vi "attributes2Variant.vi"(0 "HGF_DIMBaseType":refnum<class "HGF_DIMDataConverter.lvclass">, 2 "Parameter":variant, 3 "typeDescriptor":string, 5 "error in (no error)":errorcluster) -> (14 "HGF_DIMBaseType":refnum<class "HGF_DIMDataConverter.lvclass">, 16 "rawData":variant, 19 "error out":errorcluster)   [LabVIEW 2012, in "HGF_DIM.lvlib" / "HGF_DIMDataConverter.lvclass"]
doc: "Convert variant attributes Pn, n=0,1,2,... to raw data value of variant."
uses:
  HGF_DIMDataConverter.lvclass
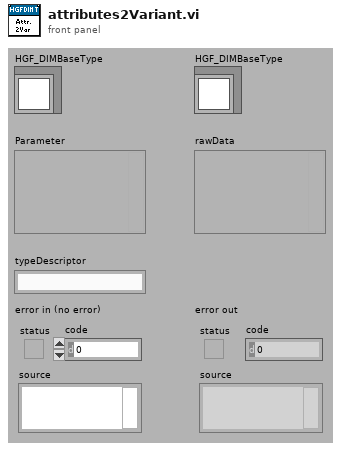
[diagram p1: front panel]
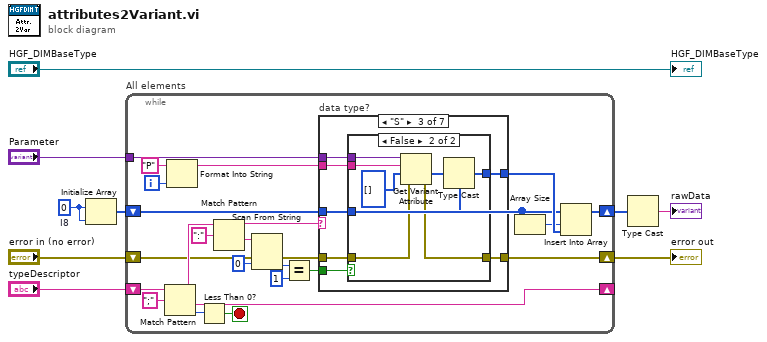
[diagram p0: block diagram]
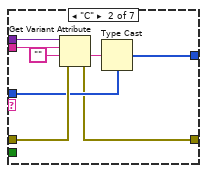
[diagram p3: hidden frame]
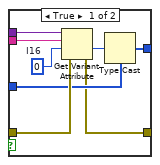
[diagram p4: hidden frame]
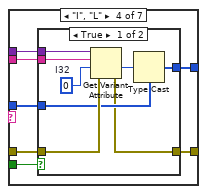
[diagram p5: hidden frame]
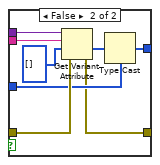
[diagram p6: hidden frame]
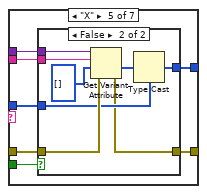
[diagram p7: hidden frame]
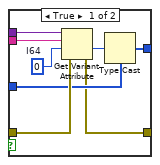
[diagram p8: hidden frame]
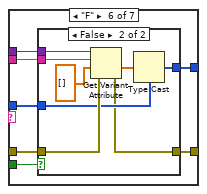
[diagram p9: hidden frame]
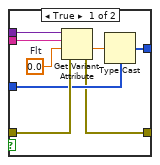
[diagram p10: hidden frame]
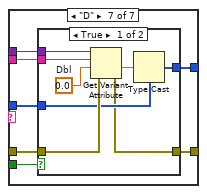
[diagram p11: hidden frame]
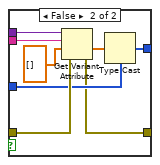
[diagram p12: hidden frame]
diagram:
  w5 = 0  # I8
  n1 = Initialize Array(w5, w5) -> (w4:i32[])
  n2 = while "All elements" {
    shift-right: [w31] -> _
    shift-left: "typeDescriptor" -> [w33]
    shift-right: [w15] -> w3
    shift-left: w4 -> [w10]
    shift-right: [w18] -> w1
    shift-left: "error in (no error)" -> [w20]
    tunnel: "Parameter" -> [w17]
    i -> [w25]
    stop <- w30 stop-if-true
    n3 = Match Pattern(string=w33, regular expression=";") -> (before substring=w28:string, after substring=w31:string, offset past match=w29:i32)  [unwired: 2 out]
    n4 = Format Into String(initial string="P", w25) -> (resulting string=w24:string)  [unwired: 2 in, 1 out]
    n5 = Less Than 0?(x=w29) -> (x < 0?=w30:bool)
    n6 = Match Pattern(string=w28, regular expression=":") -> (before substring=w23:string, after substring=w21:string)  [unwired: 3 out]
    n7 = Scan From String(input string=w21, error in=w20, default 1=0 ("default value 1")) -> (error out=w19:errorcluster, output 1=w14:i32)  [unwired: 2 in, 2 out]
    n8 = Equal?(x=w14, y=1) -> (x = y?=w12:bool)
    n9 = case "data type?" shown="\"S\"" w23 {
      tunnel: w24 -> [_ w40 w47 w70 w93 w116 w139]
      tunnel: w19 -> [w34 w41 w48 w71 w94 w117 w140]
      tunnel: [w34 w35 w44 w67 w90 w113 w136] -> w18
      tunnel: w17 -> [_ w42 w49 w72 w95 w118 w141]
      tunnel: w10 -> [_ w37 w46 w69 w92 w115 w138]
      tunnel: [_ w36 w45 w68 w91 w114 w137] -> w16
      tunnel: w12 -> [_ _ w43 w66 w89 w112 w135]
      frame Default {
      }
      frame "C" {
        n10 = Get Variant Attribute(Variant=w42, name=w40, default value (empty Variant)="", error in=w41) -> (value=w38:string, error out=w35:errorcluster)  [unwired: 2 out]
        n11 = Type Cast(type=w37, x=w38) -> (*(type *) &x=w36:i32[])
      }
      frame "S" {
        n12 = case shown="False" w43 {
          tunnel: w49 -> [w57 w65]
          tunnel: w48 -> [w56 w64]
          tunnel: w47 -> [w55 w63]
          tunnel: w46 -> [w53 w61]
          tunnel: [w52 w60] -> w45
          tunnel: [w50 w59] -> w44
          frame True {
            w51 = i16 0  # I16
            n13 = Get Variant Attribute(Variant=w57, name=w55, default value (empty Variant)=w51, error in=w56) -> (value=w54:i16, error out=w50:errorcluster)  [unwired: 2 out]
            n14 = Type Cast(type=w53, x=w54) -> (*(type *) &x=w52:i32[])
          }
          frame False {
            n15 = Get Variant Attribute(Variant=w65, name=w63, default value (empty Variant)=i16[] [], error in=w64) -> (value=w62:i16[], error out=w59:errorcluster)  [unwired: 2 out]
            n16 = Type Cast(type=w61, x=w62) -> (*(type *) &x=w60:i32[])
          }
        }
      }
      frame "I", "L" {
        n17 = case shown="True" w66 {
          tunnel: w72 -> [w80 w88]
          tunnel: w71 -> [w79 w87]
          tunnel: w70 -> [w78 w86]
          tunnel: w69 -> [w76 w84]
          tunnel: [w75 w83] -> w68
          tunnel: [w73 w82] -> w67
          frame True {
            w74 = 0  # I32
            n18 = Get Variant Attribute(Variant=w80, name=w78, default value (empty Variant)=w74, error in=w79) -> (value=w77:i32, error out=w73:errorcluster)  [unwired: 2 out]
            n19 = Type Cast(type=w76, x=w77) -> (*(type *) &x=w75:i32[])
          }
          frame False {
            n20 = Get Variant Attribute(Variant=w88, name=w86, default value (empty Variant)=i32[] [], error in=w87) -> (value=w85:i32[], error out=w82:errorcluster)  [unwired: 2 out]
            n21 = Type Cast(type=w84, x=w85) -> (*(type *) &x=w83:i32[])
          }
        }
      }
      frame "X" {
        n22 = case shown="False" w89 {
          tunnel: w95 -> [w103 w111]
          tunnel: w94 -> [w102 w110]
          tunnel: w93 -> [w101 w109]
          tunnel: w92 -> [w99 w107]
          tunnel: [w98 w106] -> w91
          tunnel: [w96 w105] -> w90
          frame True {
            w97 = i64 0  # I64
            n23 = Get Variant Attribute(Variant=w103, name=w101, default value (empty Variant)=w97, error in=w102) -> (value=w100:i64, error out=w96:errorcluster)  [unwired: 2 out]
            n24 = Type Cast(type=w99, x=w100) -> (*(type *) &x=w98:i32[])
          }
          frame False {
            n25 = Get Variant Attribute(Variant=w111, name=w109, default value (empty Variant)=i64[] [], error in=w110) -> (value=w108:i64[], error out=w105:errorcluster)  [unwired: 2 out]
            n26 = Type Cast(type=w107, x=w108) -> (*(type *) &x=w106:i32[])
          }
        }
      }
      frame "F" {
        n27 = case shown="False" w112 {
          tunnel: w118 -> [w126 w134]
          tunnel: w117 -> [w125 w133]
          tunnel: w116 -> [w124 w132]
          tunnel: w115 -> [w122 w130]
          tunnel: [w121 w129] -> w114
          tunnel: [w119 w128] -> w113
          frame True {
            w120 = sgl 0.0  # Flt
            n28 = Get Variant Attribute(Variant=w126, name=w124, default value (empty Variant)=w120, error in=w125) -> (value=w123:sgl, error out=w119:errorcluster)  [unwired: 2 out]
            n29 = Type Cast(type=w122, x=w123) -> (*(type *) &x=w121:i32[])
          }
          frame False {
            n30 = Get Variant Attribute(Variant=w134, name=w132, default value (empty Variant)=sgl[] [], error in=w133) -> (value=w131:sgl[], error out=w128:errorcluster)  [unwired: 2 out]
            n31 = Type Cast(type=w130, x=w131) -> (*(type *) &x=w129:i32[])
          }
        }
      }
      frame "D" {
        n32 = case shown="True" w135 {
          tunnel: w141 -> [w149 w157]
          tunnel: w140 -> [w148 w156]
          tunnel: w139 -> [w147 w155]
          tunnel: w138 -> [w145 w153]
          tunnel: [w144 w152] -> w137
          tunnel: [w142 w151] -> w136
          frame True {
            w143 = 0.0  # Dbl
            n33 = Get Variant Attribute(Variant=w149, name=w147, default value (empty Variant)=w143, error in=w148) -> (value=w146:dbl, error out=w142:errorcluster)  [unwired: 2 out]
            n34 = Type Cast(type=w145, x=w146) -> (*(type *) &x=w144:i32[])
          }
          frame False {
            n35 = Get Variant Attribute(Variant=w157, name=w155, default value (empty Variant)=dbl[] [], error in=w156) -> (value=w154:dbl[], error out=w151:errorcluster)  [unwired: 2 out]
            n36 = Type Cast(type=w153, x=w154) -> (*(type *) &x=w152:i32[])
          }
        }
      }
    }
    n37 = Array Size(array=w10) -> (size(s)=w11:i32)
    n38 = Insert Into Array(array=w10, index=w11, new element=w16) -> (w15:i32[])
  }
  "error out" <- w1
  n39 = Type Cast(x=w3) -> (*(type *) &x=→"rawData":string)  [unwired: 1 out]
  "HGF_DIMBaseType" <- "HGF_DIMBaseType"
